vi "Set Project Ref.vi"(10 "Project Ref":refnum<vi>, 11 "CD Build Tools in":refnum<class "Project Sync Tools.lvclass">) -> (3 "CD Build Tools out":refnum<class "Project Sync Tools.lvclass">)   [LabVIEW 2019, in "Project Sync Tools.lvclass"]
uses:
  Project Sync Tools.lvclass
  Project Sync Tools.lvclass/Project Sync Tools.ctl
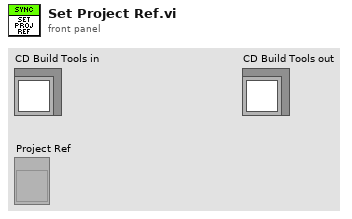
[diagram p1: front panel]
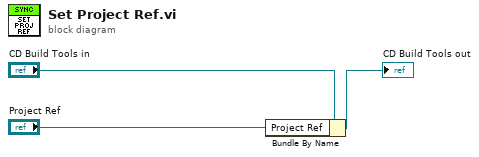
[diagram p0: block diagram]
diagram:
  n1 = Bundle By Name(cluster="CD Build Tools in", "Project Ref"="Project Ref") -> (→"CD Build Tools out":refnum<class "Project Sync Tools.lvclass">)
